vi "testing StringAndValues[] ring update.vi"() -> ()   [LabVIEW 2021]
uses:
  type-defs/stimulator configuration line cluster (type def).ctl
  type-defs/port-odor with color cluster (type def).ctl
  type-defs/port-odor ring (type def).ctl
  type-defs/odor color (type def).ctl
  type-defs/ring string and value cluster (type def).ctl
panel:
  in  "stop":bool
  in  "stim. config line":T1={"description"="", "duration, s"=0.0, "left odor"={"port-odor ring"=0, "odor color"=9}, "middle odor"={"port-odor ring"=0, "odor color"=9}, "right odor"={"port-odor ring"=0, "odor color"=9}} {"right odor"."port-odor ring" items=["off"=0, "world"=3]; "middle odor"."port-odor ring" items=["off"=0, "good"=2]; "left odor"."port-odor ring" items=["off", "helllo"]}
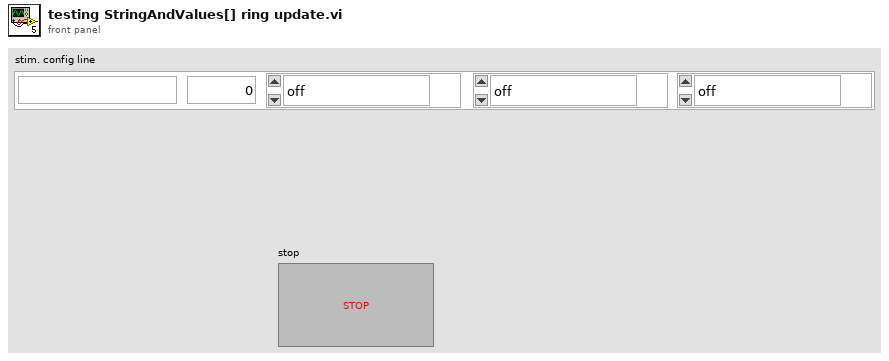
[diagram p1: front panel]
types:
  T1 = typedef "stimulator configuration line cluster (type def).ctl" = cluster{"description":string, "duration, s":dbl, "left odor":T2, "middle odor":T2, "right odor":T2}
  T2 = typedef "port-odor with color cluster (type def).ctl" = cluster{"port-odor ring":T3, "odor color":T4}
  T3 = typedef "port-odor ring (type def).ctl" = u16
  T4 = typedef "odor color (type def).ctl" = u16
  T5 = typedef "ring string and value cluster (type def).ctl" = cluster{"String":string, "Value":u16}
  T6 = cluster{"description string":refnum<vi>, "duration, s numeric":refnum<vi>, "port-odor & color cluster []":refnum<vi>[], "port-odor ring []":refnum<vi>[], "odor color ring []":refnum<vi>[]}
  T7 = typedef "LVStringsAndValuesArrayTypeDef_U16.ctl" = cluster{"String":string, "Value":u16}[]
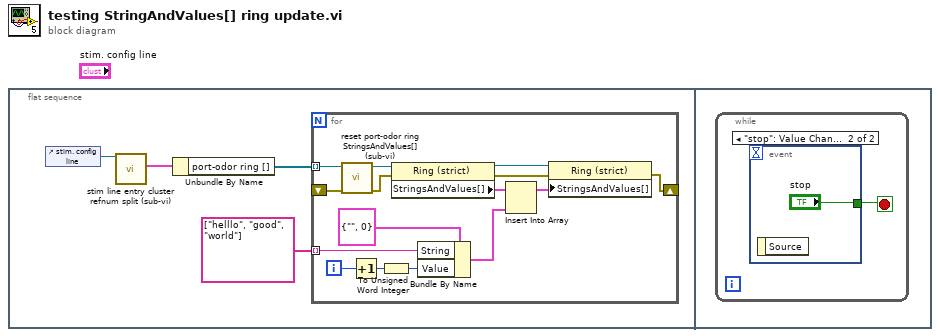
[diagram p0: block diagram]
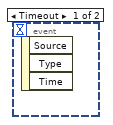
[diagram p2: hidden frame]
diagram:
  n1 = flat-sequence {
    frame #0 {
      n2 = control-ref of="stim. config line"() -> (w3:refnum<vi>)
      n3 = call "stim line entry cluster refnum split (sub-vi).vi"("stim. config line cluster refnum"=w3) -> ("element refnum cluster"=w2:T6)  [unwired: 8 in, 2 out]
      n4 = Unbundle By Name(w2) -> ("port-odor ring []"=w1:refnum<vi>[])
      n5 = for {
        tunnel: string[] ["helllo", "good", "world"] -> [w17] mode=indexing
        shift-right: [w7] -> _
        shift-left: _ -> [w6]
        tunnel: w1 -> [w5] mode=indexing
        i -> [w18]
        n6 = call "reset port-odor ring StringsAndValues[] (sub-vi).vi"("error in (no error)"=w6, "port-odor ring refnum"=w5) -> ("error out"=w9:errorcluster, "port-odor ring refnum out"=w13:refnum<vi>)  [unwired: 8 in]
        n7 = Increment(x=w18) -> (x+1=w14:i32)
        n8 = To Unsigned Word Integer(number=w14) -> (unsigned 16bit integer=w11:u16)
        n9 = property class="Ring (strict)"(reference=w13, error in=w9) -> (reference out=w15:refnum<vi>, error out=w8:errorcluster, "StringsAndValues[]"=w19:T7)
        n10 = Bundle By Name(cluster=T5 {"String"="", "Value"=0} ("output cluster"), "String"=w17, "Value"=w11) -> (w10:T5)
        n11 = Insert Into Array(array=w19, new element=w10) -> (w16:T7)  [unwired: 1 in]
        n12 = property class="Ring (strict)"(reference=w15, error in=w8, "StringsAndValues[]"=w16) -> (error out=w7:errorcluster)  [unwired: 1 out]
      }
    }
    frame #1 {
      n13 = while {
        stop <- w20 stop-if-true
        n14 = event shown="[1] \"stop\": Value Change" {
          selector: _ -> [_ _]
          dyn-events: _ -> [_ _]
          timeout: _ -> [_ _]
          tunnel: [_ "stop"] -> w20
          event Timeout {
            n15 = event-data() -> ()  [unwired: 1 in, 3 out]
          }
          event "stop": Value Change {
            n16 = event-data() -> ()  [unwired: 1 in, 1 out]
          }
        }
      }
    }
  }
